vi "WriteFile.vi"(0 "object in":refnum<class "File.lvclass">, 2 "Data In":T1, 5 "error in (no error)":errorcluster) -> (14 "object out":refnum<class "File.lvclass">, 19 "error out":errorcluster)   [LabVIEW 2021, in "File.lvclass"]
uses:
  File.lvclass
  File.lvclass/File.ctl
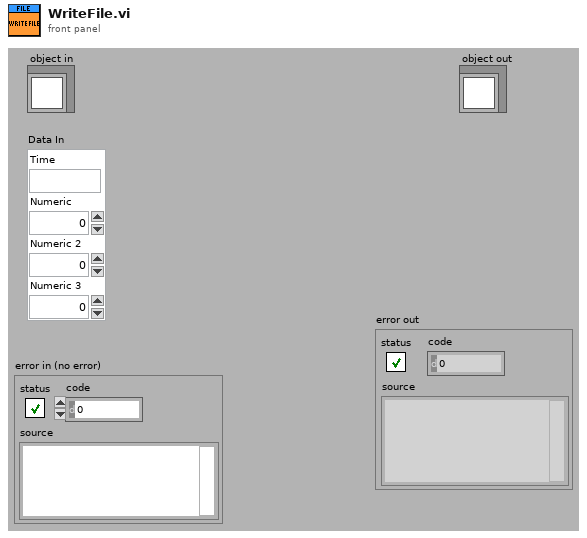
[diagram p1: front panel]
types:
  T1 = cluster{"Time":string, "Numeric":dbl, "Numeric 2":dbl, "Numeric 3":dbl}
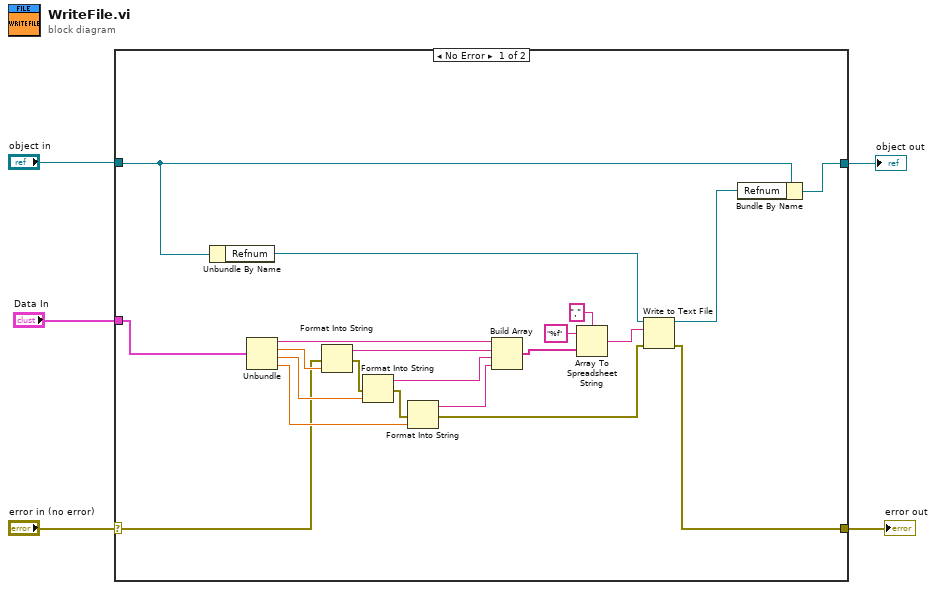
[diagram p0: block diagram]
diagram:
  n1 = case shown="No Error" "error in (no error)" {
    selector: "error in (no error)" -> [w13 w28]
    tunnel: [w6 w28] -> w4
    tunnel: [w25 w27] -> w2
    tunnel: "object in" -> [w26 w27]
    tunnel: "Data In" -> [w24 _]
    frame No Error {
      n2 = Unbundle By Name(w26) -> ("Refnum"=w19:refnum<file>)
      n3 = Unbundle(w24) -> ("Time"=w18:string, "Numeric"=w16:dbl, "Numeric 2"=w15:dbl, "Numeric 3"=w14:dbl)
      n4 = Format Into String(error in=w13, w16) -> (resulting string=w10:string, error out=w12:errorcluster)  [unwired: 2 in]
      n5 = Format Into String(error in=w12, w15) -> (resulting string=w9:string, error out=w11:errorcluster)  [unwired: 2 in]
      n6 = Format Into String(error in=w11, w14) -> (resulting string=w8:string, error out=w7:errorcluster)  [unwired: 2 in]
      n7 = Build Array(w18, w10, w9, w8) -> (w17:string[])
      n8 = Array To Spreadsheet String(delimiter (Tab)=",", array=w17, 3:"%f" ("format string")) -> (spreadsheet string=w21:string)
      n9 = Write to Text File(file (use dialog)=w19, text=w21, error in=w7) -> (refnum out=w20:refnum<file>, error out=w6:errorcluster)  [unwired: 1 in, 1 out]
      n10 = Bundle By Name(cluster=w26, "Refnum"=w20) -> (w25:refnum<class "File.lvclass">)
    }
    frame Error {
    }
  }
  "error out" <- w4
  "object out" <- w2
